vi "Untitled 3.vi"() -> ()   [LabVIEW 2021]
uses:
  <vilib>/Analysis/NI_AALBase.lvlib
panel:
  out "Variance":dbl
  out "Standard Deviation":dbl format="%#_2g"
  out "Mean":dbl format="%#_1f"
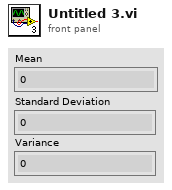
[diagram p1: front panel]
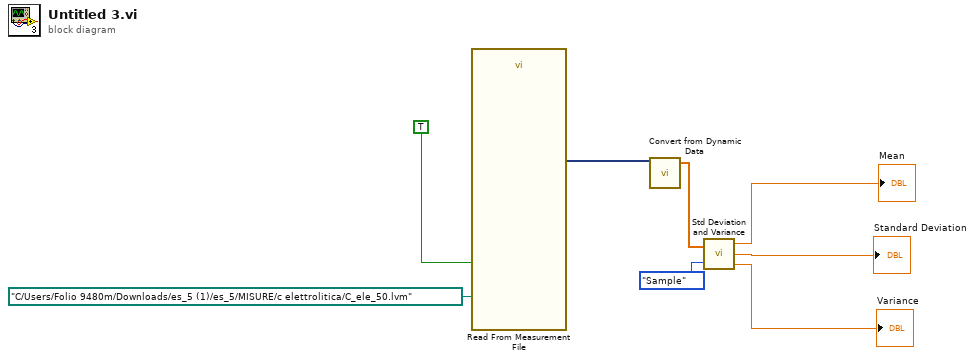
[diagram p0: block diagram]
diagram:
  n1 = call "Read From Measurement File"("Filename"=path "C:/Users/Folio 9480m/Downloads/es_5 (1)/es_5/MISURE/c elettrolitica/C_ele_50.lvm", "Enable"=TRUE) -> ("Signals"=w8:dynamicdata)  [unwired: 4 in, 5 out]
  n2 = call "Convert from Dynamic Data"("Dynamic Data Type"=w8) -> ("Array"=w7:dbl[])  [unwired: 3 in]
  n3 = call <vilib>:"Std Deviation and Variance.vi"("X"=w7, "Weighting (Sample)"=enum16{"Sample", "Population"}."Sample") -> ("mean"=→"Mean":dbl, "standard deviation"=→"Standard Deviation":dbl, "variance"=→"Variance":dbl)
